vi "initializeDefaultStyle.vi"(8 "error in (no error)":errorcluster, 11 "Figure in":refnum<class "Figure.lvclass">) -> (0 "error out":errorcluster, 3 "Figure out":refnum<class "Figure.lvclass">)   [LabVIEW 2017, in "Styles.lvlib" / "Figure.lvclass"]
uses:
  Figure.lvclass
  C:/Users/Neo/Desktop/Dev_Tools_BR/LabVIEW_NPOI/src/Styles/Style/Style.lvclass
  Alignment--ring.ctl
  Style/Style.lvclass
  Styles.lvlib
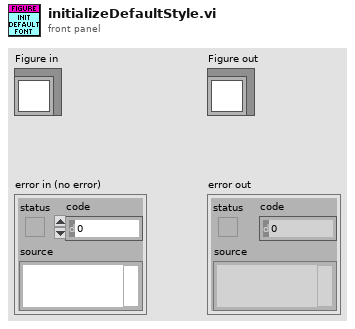
[diagram p1: front panel]
types:
  T1 = typedef "Styles.lvlib/Alignment--ring.ctl" = i32
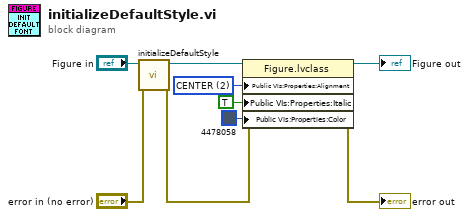
[diagram p0: block diagram]
diagram:
  w3 = T1 2 items=["LEFT"=1, "CENTER"=2, "RIGHT"=3, "BOTH"=4, "MEDIUM_KASHIDA"=5, "DISTRIBUTE"=6, "NUM_TAB"=7, "HIGH_KASHIDA"=8, "LOW_KASHIDA"=9, "THAI_DISTRIBUTE"=10] ("Font:Alignment")
  n1 = call-parent "initializeDefaultStyle.vi"("error in (no error)"="error in (no error)", "Style in"="Figure in") -> ("error out"=w5:errorcluster, "Style out"=w9:refnum<class "Figure.lvclass">)  [unwired: 8 in]
  n2 = property class="Figure.lvclass"(reference=w9, error in=w5, "Public VIs:Properties:Alignment"=w3, "Public VIs:Properties:Italic"=TRUE ("Font:Italic"), "Public VIs:Properties:Color"=u32 4478058 ("Font:Color:Color")) -> (reference out=→"Figure out":refnum<class "Figure.lvclass">, error out=→"error out":errorcluster)
